vi "Parse Contained Variables.vi"(8 "Error in":errorcluster caption="Error in (no error)", 11 "String":string="${case${select}.addr}+${protocol}://${ip}:${port}") -> (0 "Error out":errorcluster, 3 "Contained Variables":string[](array[string]))   [LabVIEW 2017, in "CSM Shared.lvlib"]
uses:
  CSM Shared.lvlib
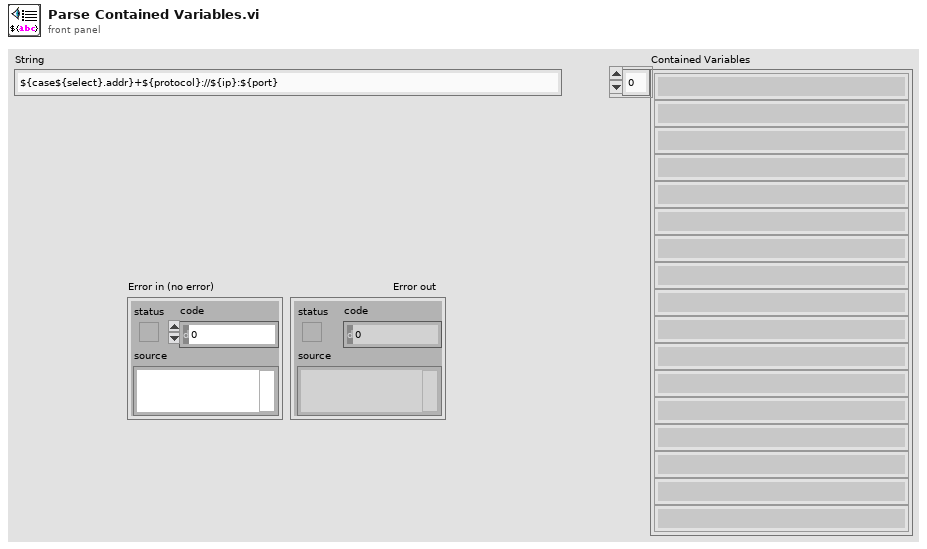
[diagram p1: front panel]
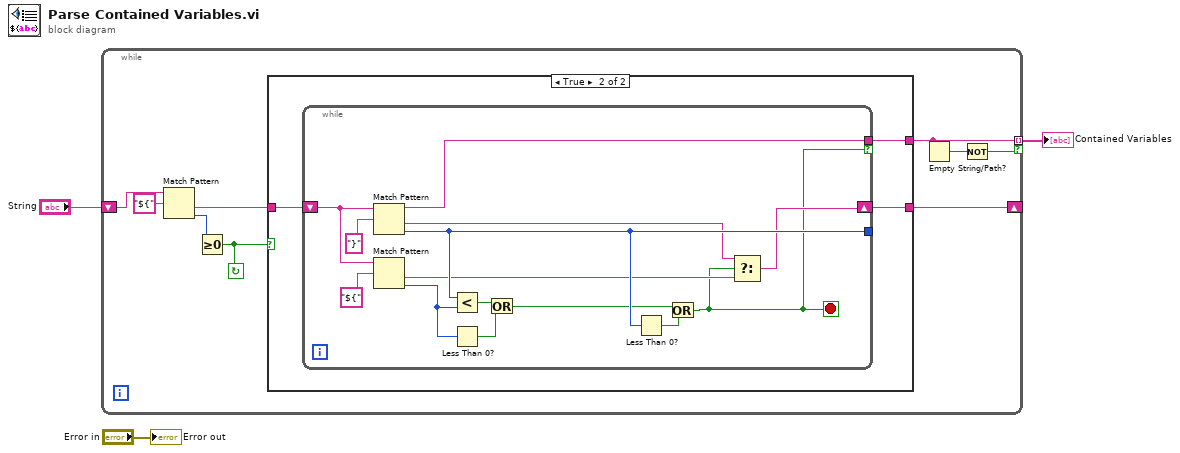
[diagram p0: block diagram]
diagram:
  n1 = while {
    shift-right: [w11] -> _
    shift-left: "String" -> [w12]
    tunnel: [w8] -> w2 mode=indexing if=w7
    stop <- w10 continue-if-true
    n2 = Match Pattern(string=w12, regular expression="${") -> (after substring=w4:string, offset past match=w5:i32)  [unwired: 1 in, 2 out]
    n3 = Greater Or Equal To 0?(x=w5) -> (x >= 0?=w10:bool)
    n4 = case shown="True" w10 {
      tunnel: w4 -> [w13 w16]
      tunnel: [w13 w15] -> w11
      tunnel: [_ w14] -> w8
      frame False {
      }
      frame True {
        n5 = while {
          tunnel: [w24] -> _
          shift-right: [w19] -> w15
          shift-left: w16 -> [w28]
          tunnel: [w18] -> w14 if=w17
          stop <- w17 stop-if-true
          n6 = Match Pattern(string=w28, regular expression="}") -> (before substring=w18:string, after substring=w20:string, offset past match=w24:i32)  [unwired: 1 in, 1 out]
          n7 = Match Pattern(string=w28, regular expression="${") -> (after substring=w21:string, offset past match=w25:i32)  [unwired: 1 in, 2 out]
          n8 = Less?(x=w24, y=w25) -> (x < y?=w27:bool)
          n9 = Less Than 0?(x=w25) -> (x < 0?=w22:bool)
          n10 = Or(x=w27, y=w22) -> (x .or. y?=w23:bool)
          n11 = Less Than 0?(x=w24) -> (x < 0?=w26:bool)
          n12 = Or(x=w23, y=w26) -> (x .or. y?=w17:bool)
          n13 = Select(t=w20, s=w17, f=w21) -> (s? t:f=w19:string)
        }
      }
    }
    n14 = Empty String/Path?(string/path=w8) -> (empty?=w9:bool)
    n15 = Not(x=w9) -> (.not. x?=w7:bool)
  }
  "Contained Variables" <- w2
  "Error out" <- "Error in"
